vi "校准设置页.vi"() -> ()   [LabVIEW 2016, in "斯坦道氨氮.lvlib"]
uses:
  <vilib>/Analysis/6fits.llb/Curve Fitting Criteria.ctl
  <vilib>/Analysis/NI_AALPro.lvlib
  <vilib>/ptbypt/NI_PtbyPt.lvlib
panel:
  out "刷新时间":string
  out "校准状态":T1(ring)
  out "模型刷新":bool
  in  "校准按钮":T2(radio)
  in  "校准导入":bool
  in  "辅助计算":bool
  in  "曲线模型":T3={"标液浓度1"=0.0, "测量吸光度1"=0.0, "样品1启用"=FALSE, "标液浓度2"=0.0, "测量吸光度2"=0.0, "样品2启用"=FALSE, "标液浓度3"=0.0, "测量吸光度3"=0.0, "样品3启用"=FALSE, "标液浓度4"=0.0, "测量吸光度4"=0.0, "样品4启用"=FALSE, "标液浓度5"=0.0, "测量吸光度5"=0.0, "样品5启用"=FALSE, "模型"=enum."线性", "精度"=4.0, "XY图"=[], "拟合公式"="", "r^2"=0.0, "标样一校准时间"=timestamp(0 s since 1904-01-01), "标样二校准时间"=timestamp(0 s since 1904-01-01), "标样三校准时间"=timestamp(0 s since 1904-01-01), "标样四校准时间"=timestamp(0 s since 1904-01-01), "标样五校准时间"=timestamp(0 s since 1904-01-01), "二次方程"={"c"=0.0, "x"=0.0, "x^2"=0.0}, "标定时间"=timestamp(0 s since 1904-01-01)} {"标定时间" format="%<%m/%d/%y %H:%M:%S>T"; "标样五校准时间" format="%<%m/%d/%y %H:%M:%S>T"; "标样四校准时间" format="%<%m/%d/%y %H:%M:%S>T"; "标样三校准时间" format="%<%m/%d/%y %H:%M:%S>T"; "标样二校准时间" format="%<%m/%d/%y %H:%M:%S>T"; "标样一校准时间" format="%<%m/%d/%y %H:%M:%S>T"; "r^2" format="%.7f"; "测量吸光度5" format="%#.6f"; "测量吸光度4" format="%#.6f"; "测量吸光度3" format="%#.6f"; "测量吸光度2" format="%#.6f"; "测量吸光度1" format="%#.6f"}
  in  "测量模式":T4(ring)
  in  "参数下拉列表":u16(ring)
  in  "量程下拉列表":enum16{"低量程", "高量程"}(ring)
  # "校准时间"
  # "标液浓度"
  # "吸光值显示"
  # "标液一"
  # "标液二"
  # "标液三"
  # "零点"
  # "跨度"
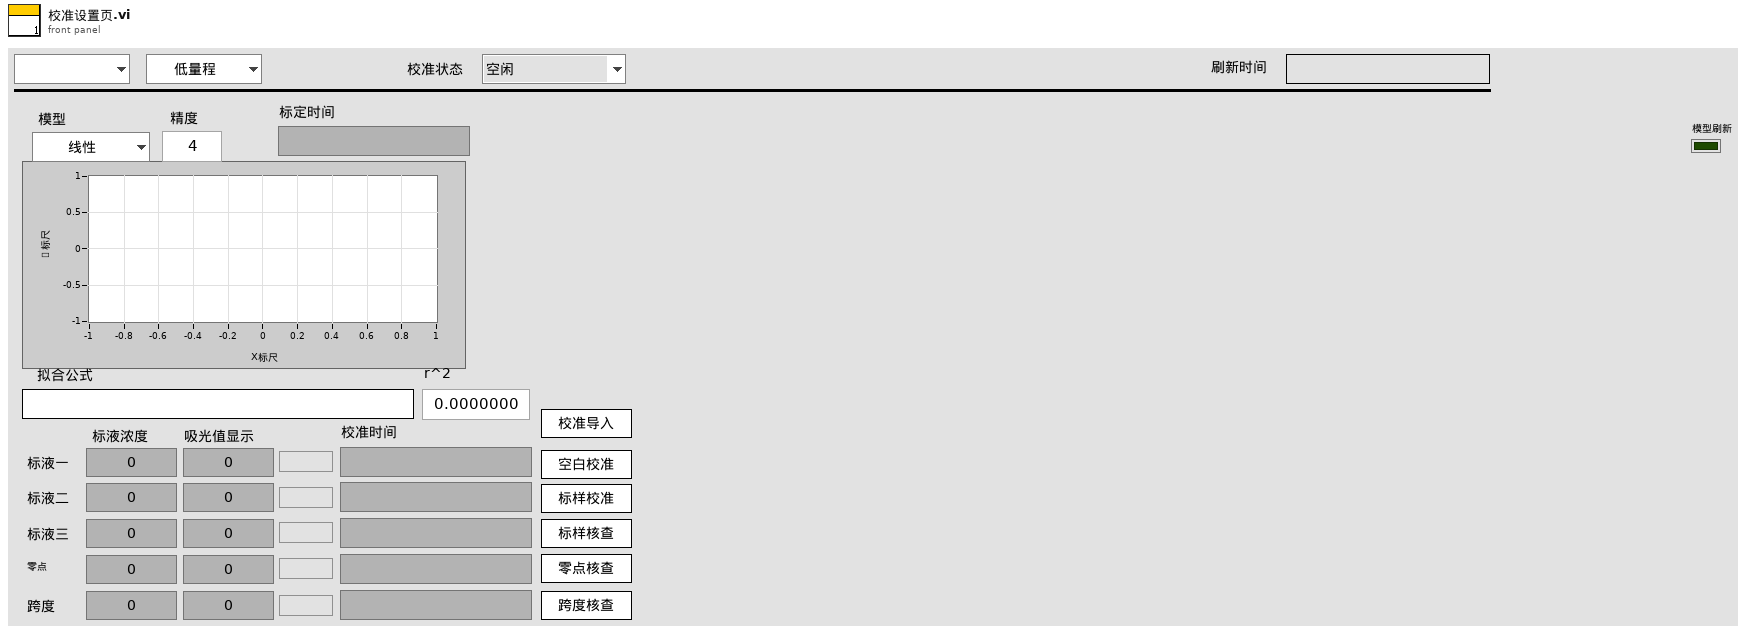
[diagram p1: front panel]
types:
  T1 = enum16{"空闲", "初始化", "校准启动", "校准运行中", "测试结束", "获取校准数据", "填充校准数据", "流程结束"}
  T2 = enum32{"未选择", "空白校准", "标样校准", "标样核查", "零点核查", "跨度核查"}
  T3 = cluster{"标液浓度1":dbl, "测量吸光度1":dbl, "样品1启用":bool, "标液浓度2":dbl, "测量吸光度2":dbl, "样品2启用":bool, "标液浓度3":dbl, "测量吸光度3":dbl, "样品3启用":bool, "标液浓度4":dbl, "测量吸光度4":dbl, "样品4启用":bool, "标液浓度5":dbl, "测量吸光度5":dbl, "样品5启用":bool, "模型":enum32{"线性", "多项式"}, "精度":dbl, "XY图":cluster{"X Values":dbl[], "Y Values":dbl[]}[], "拟合公式":string, "r^2":dbl, "标样一校准时间":timestamp, "标样二校准时间":timestamp, "标样三校准时间":timestamp, "标样四校准时间":timestamp, "标样五校准时间":timestamp, "二次方程":cluster{"c":dbl, "x":dbl, "x^2":dbl}, "标定时间":timestamp}
  T4 = enum16{"跨度核查", "水样测量", "零点核查", "标样核查", "加标回收", "快捷测试", "空白校准", "标样校准"}
  T5 = typedef "LVStringsAndValuesArrayTypeDef_U16.ctl" = cluster{"String":string, "Value":u16}[]
  T6 = enum8{"Enabled", "Disabled", "Disabled and Grayed Out"}
  T7 = cluster{"标液浓度1":dbl, "测量吸光度1":dbl, "样品1启用":bool, "标液浓度2":dbl, "测量吸光度2":dbl, "样品2启用":bool, "标液浓度3":dbl, "测量吸光度3":dbl, "样品3启用":bool, "标液浓度4":dbl, "测量吸光度4":dbl, "样品4启用":bool, "标液浓度5":dbl, "测量吸光度5":dbl, "样品5启用":bool, "模型":enum32{"线性", "多项式"}, "精度":dbl, "XY图":cluster{"X Values":dbl[], "Y Values":dbl[]}[], "拟合公式":string, "r^2":dbl, "标样一校准时间":timestamp, "标样二校准时间":timestamp, "标样三校准时间":timestamp, "标样四校准时间":timestamp, "标样五校准时间":timestamp, "二次方程":cluster{"c":dbl, "x":dbl, "x^2":dbl}, "标定时间":timestamp}[][]
  T8 = typedef "NI_AALPro.lvlib/Curve Fitting Criteria.ctl" = u16
  T9 = enum32{"Bad", "Idle", "Run top level", "Running"}
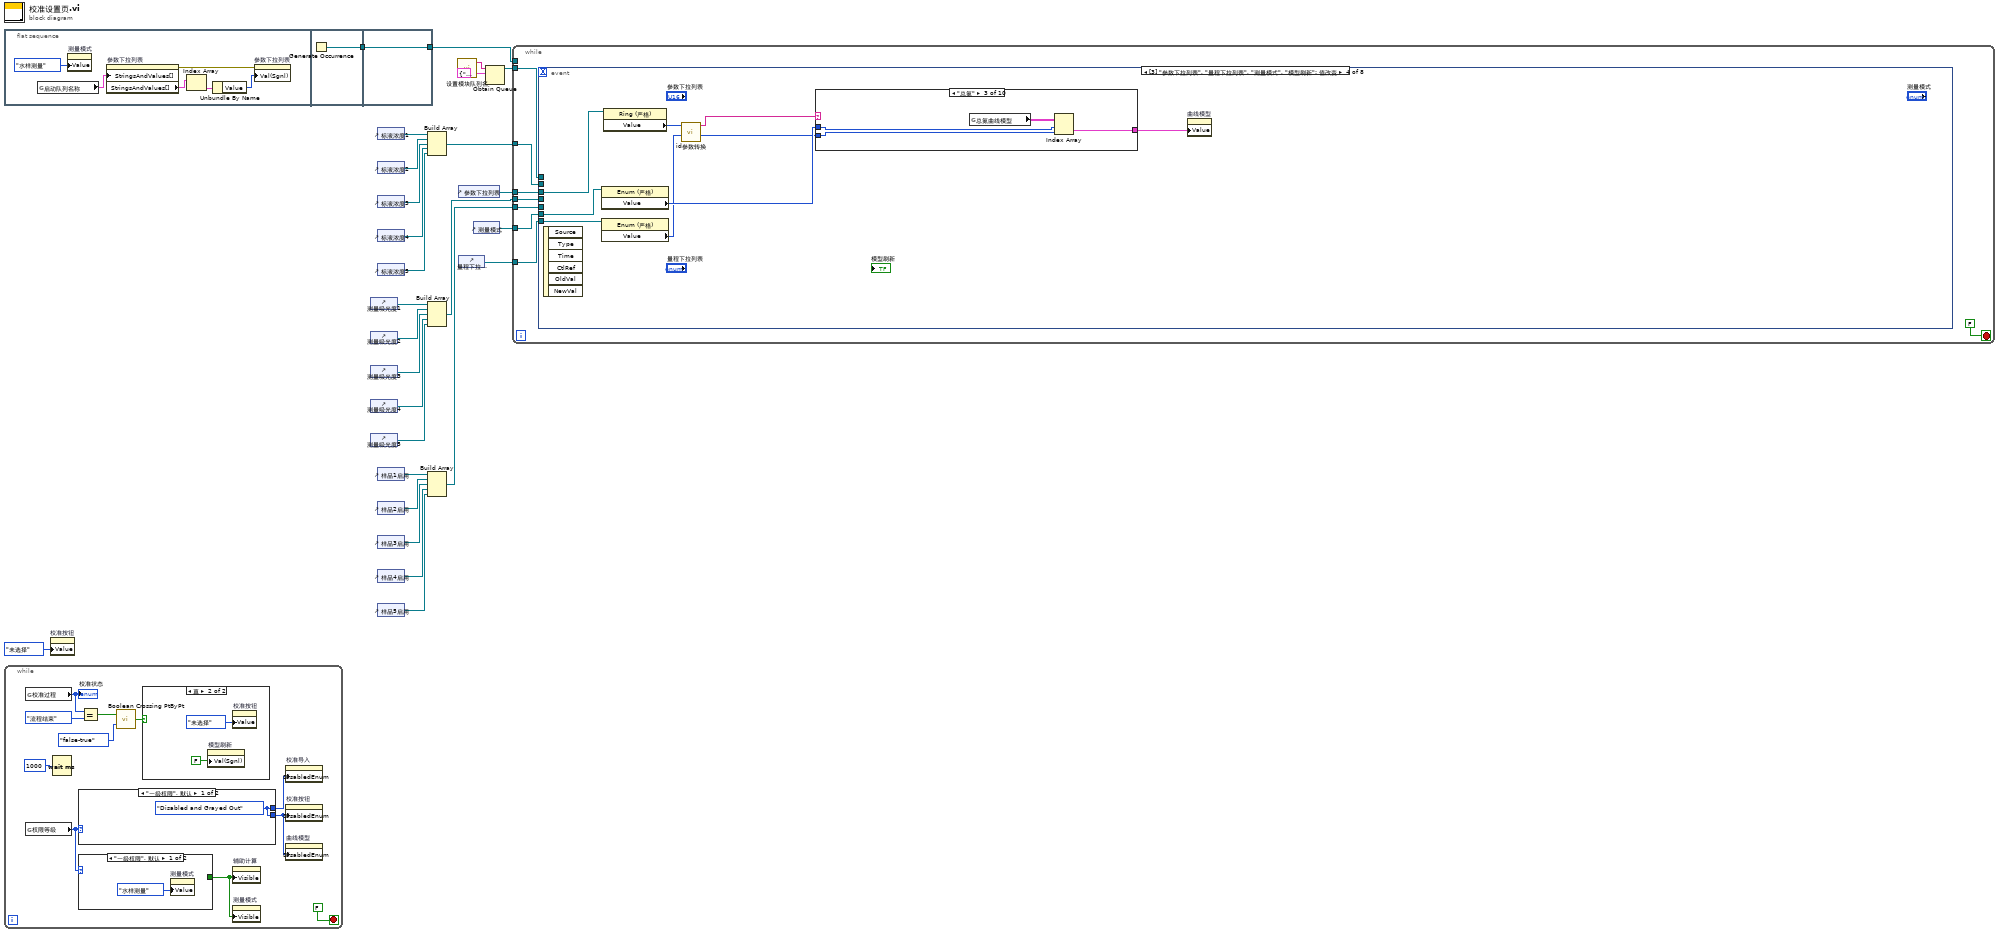
[diagram p0: block diagram]
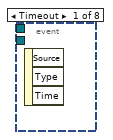
[diagram p2: hidden frame]
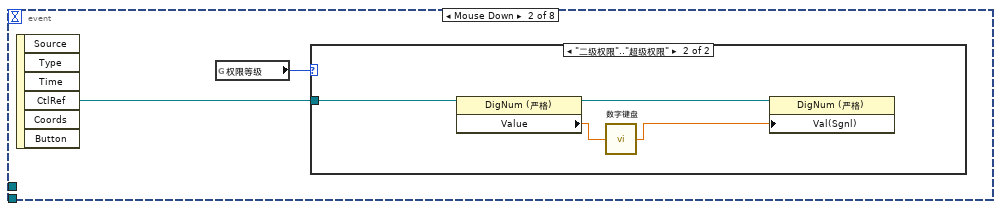
[diagram p3: hidden frame]
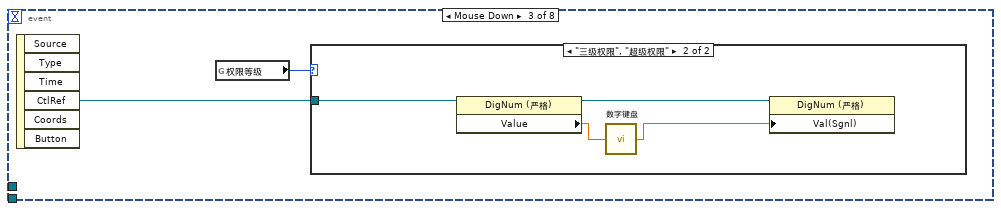
[diagram p5: hidden frame]
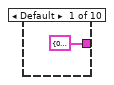
[diagram p7: hidden frame]
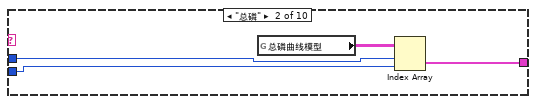
[diagram p8: hidden frame]
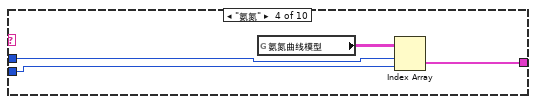
[diagram p9: hidden frame]
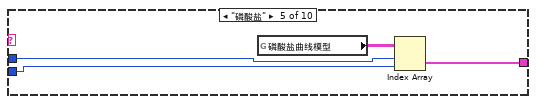
[diagram p10: hidden frame]
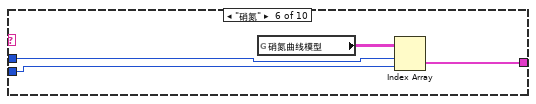
[diagram p11: hidden frame]
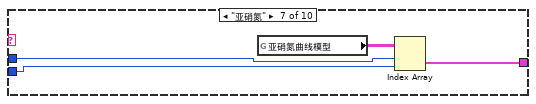
[diagram p12: hidden frame]
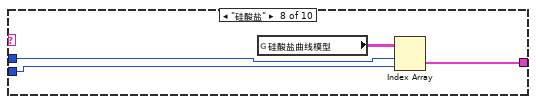
[diagram p13: hidden frame]
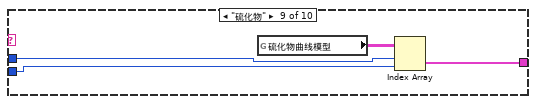
[diagram p14: hidden frame]
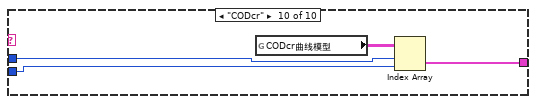
[diagram p15: hidden frame]
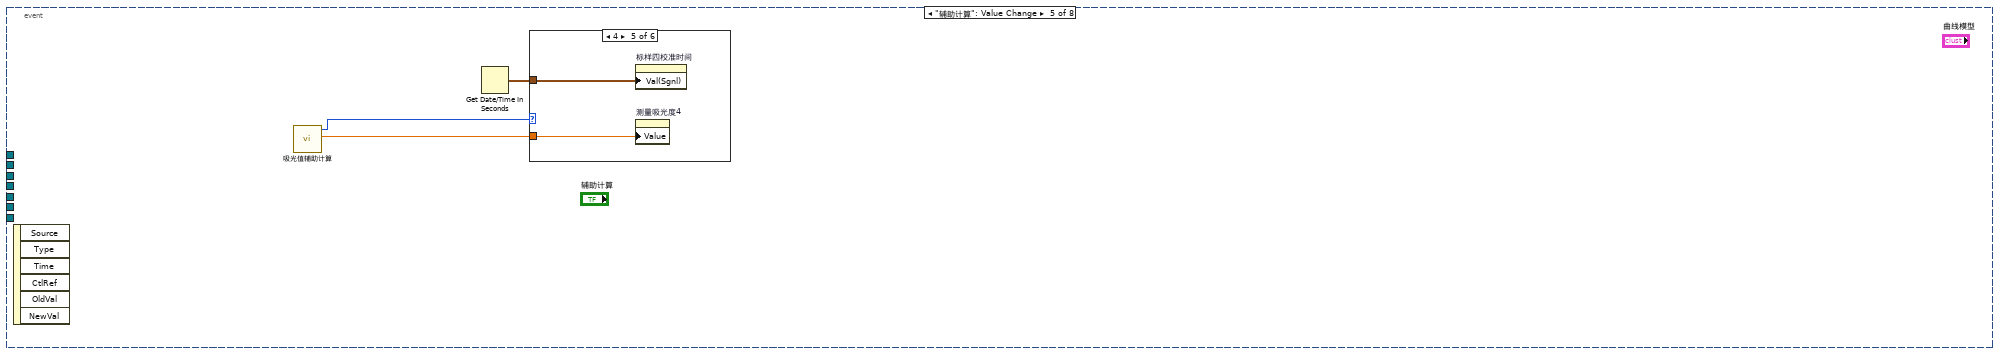
[diagram p16: hidden frame]
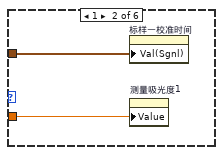
[diagram p18: hidden frame]
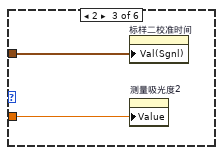
[diagram p19: hidden frame]
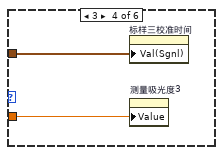
[diagram p20: hidden frame]
diagram:
  n1 = flat-sequence {
    tunnel: [w34] -> w27
    tunnel: [w35] -> w26
    tunnel: w27 -> [w35]
    frame #0 {
      n2 = global read "总磷总氮断电保存全局变量.vi" "启动队列名称"() -> (w29:cluster{"String":string, "Value":u16}[])
      n3 = property on="测量模式" class="Enum (严格)"("Value"=T4."水样测量" ("测量模式")) -> ()  [unwired: 2 in, 2 out]
      n4 = property on="参数下拉列表" class="Ring (严格)"("StringsAndValues[]"=w29) -> (error out=w32:errorcluster, "StringsAndValues[]"=w30:T5)  [unwired: 2 in, 1 out]
      n5 = Index Array(array=w30) -> (element=w31:cluster{"String":string, "Value":u16})  [unwired: 1 in]
      n6 = Unbundle By Name(w31) -> ("Value"=w33:u16)
      n7 = property on="参数下拉列表" class="Ring (严格)"(error in=w32, "Val(Sgnl)"=w33) -> ()  [unwired: 1 in, 2 out]
    }
    frame #1 {
      n8 = Generate Occurrence() -> (w34:refnum<k4>)
    }
    frame #2 {
    }
  }
  n9 = while {
    stop <- FALSE stop-if-true
    n10 = global read "VAR总磷总氮全局变量.vi" "校准过程"() -> (w37:T1)
    "校准状态" <- w37
    n11 = global read "VAR总磷总氮全局变量.vi" "权限等级"() -> (w43:enum16{"一级权限", "二级权限", "三级权限", "超级权限"})
    n12 = Wait (ms)(milliseconds to wait=u32 1000 ("等待时间（毫秒）")) -> ()  [unwired: 1 out]
    n13 = case shown="\"一级权限\", 默认" w43 {
      tunnel: [w51 w52] -> w41
      tunnel: [w51 w52] -> w44
      frame "一级权限", Default {
        w51 = T6."Disabled and Grayed Out" ("禁用")
      }
      frame "二级权限".."超级权限" {
        w52 = T6."Enabled" ("禁用")
      }
    }
    n14 = case shown="\"一级权限\", 默认" w43 {
      tunnel: [_ TRUE ("可见")] -> w42
      frame "一级权限", Default {
        n15 = property on="测量模式" class="Enum (严格)"("Value"=T4."水样测量" ("测量模式")) -> ()  [unwired: 2 in, 2 out]
      }
      frame "三级权限", "超级权限" {
      }
    }
    n16 = Equal?(x=w37, y=T1."流程结束" ("校准过程")) -> (x = y?=w40:bool)
    n17 = call <vilib>:"Boolean Crossing PtByPt.vi"("direction"=enum16{"either", "false-true", "true-false"}."false-true", "input"=w40) -> ("crossing"=w38:bool)  [unwired: 1 in]
    n18 = case shown="真" w38 {
      frame False {
      }
      frame True {
        n19 = property on="模型刷新" class="Bool (严格)"("Val(Sgnl)"=FALSE ("值(信号)")) -> ()  [unwired: 2 in, 2 out]
        n20 = property on="校准按钮" class="RadioBtnsControl (严格)"("Value"=T2."未选择" ("校准按钮")) -> ()  [unwired: 2 in, 2 out]
      }
    }
    n21 = property on="辅助计算" class="Bool"("Visible"=w42) -> ()  [unwired: 2 in, 2 out]
    n22 = property on="测量模式" class="Enum (严格)"("Visible"=w42) -> ()  [unwired: 2 in, 2 out]
    n23 = property on="校准导入" class="Bool"("DisabledEnum"=w44) -> ()  [unwired: 2 in, 2 out]
    n24 = property on="校准按钮" class="RadioBtnsControl (严格)"("DisabledEnum"=w41) -> ()  [unwired: 2 in, 2 out]
    n25 = property on="曲线模型" class="Clust (严格)"("DisabledEnum"=w41) -> ()  [unwired: 2 in, 2 out]
  }
  n26 = property on="校准按钮" class="RadioBtnsControl (严格)"("Value"=T2."未选择" ("校准按钮")) -> ()  [unwired: 2 in, 2 out]
  n27 = control-ref of="测量吸光度1"() -> (w15:refnum<vi>)
  n28 = control-ref of="测量吸光度2"() -> (w16:refnum<vi>)
  n29 = control-ref of="测量吸光度3"() -> (w17:refnum<vi>)
  n30 = control-ref of="测量吸光度4"() -> (w18:refnum<vi>)
  n31 = control-ref of="测量吸光度5"() -> (w19:refnum<vi>)
  n32 = control-ref of="标液浓度1"() -> (w13:refnum<vi>)
  n33 = control-ref of="标液浓度2"() -> (w12:refnum<vi>)
  n34 = control-ref of="标液浓度3"() -> (w11:refnum<vi>)
  n35 = control-ref of="标液浓度4"() -> (w10:refnum<vi>)
  n36 = control-ref of="标液浓度5"() -> (w9:refnum<vi>)
  n37 = control-ref of="样品1启用"() -> (w25:refnum<vi>)
  n38 = control-ref of="样品2启用"() -> (w24:refnum<vi>)
  n39 = control-ref of="样品3启用"() -> (w23:refnum<vi>)
  n40 = control-ref of="样品4启用"() -> (w22:refnum<vi>)
  n41 = control-ref of="样品5启用"() -> (w21:refnum<vi>)
  n42 = Build Array(w13, w12, w11, w10, w9) -> (w8:refnum<vi>[])
  n43 = Build Array(w15, w16, w17, w18, w19) -> (w14:refnum<vi>[])
  n44 = Build Array(w25, w24, w23, w22, w21) -> (w20:refnum<vi>[])
  n45 = call "设置模块队列名.vi"() -> ("Msg"=w6:string)  [unwired: 5 in]
  n46 = control-ref of="参数下拉列表"() -> (w3:refnum<vi>)
  n47 = control-ref of="量程下拉列表"() -> (w1:refnum<vi>)
  n48 = control-ref of="测量模式"() -> (w2:refnum<vi>)
  n49 = Obtain Queue(name (unnamed)=w6, element data type=cluster{"命令":string, "data":variant} {"命令"="", "data"=variant}) -> (queue out=w5:refnum<queue>)  [unwired: 3 in, 2 out]
  n50 = while {
    tunnel: w26 -> [_]
    tunnel: w3 -> [w59]
    tunnel: w20 -> [w58]
    tunnel: w14 -> [w57]
    tunnel: w8 -> [w56]
    tunnel: w2 -> [w55]
    tunnel: w1 -> [w54]
    tunnel: w5 -> [w53]
    stop <- FALSE stop-if-true
    n51 = event shown="[3] \"参数下拉列表\", \"量程下拉列表\", \"测量模式\", \"模型刷新\": 值改变" {
      selector: _ -> [_ _ _ _ _ _ _ _]
      dyn-events: _ -> [_ _ _ _ _ _ _ _]
      timeout: _ -> [_ _ _ _ _ _ _ _]
      tunnel: w59 -> [_ _ _ w79 _ w143 w189 w278]
      tunnel: w58 -> [_ _ _ _ _ _ w193 _]
      tunnel: w57 -> [_ _ _ _ _ _ w192 _]
      tunnel: w56 -> [_ _ _ _ _ _ w191 _]
      tunnel: w55 -> [_ _ _ w77 _ w141 w187 w273]
      tunnel: w54 -> [_ _ _ w76 _ w139 w185 w277]
      tunnel: w53 -> [_ _ _ _ _ _ _ w279]
      event Timeout {
        n52 = event-data() -> ()  [unwired: 1 in, 3 out]
      }
      event "曲线模型.标液浓度1", "曲线模型.标液浓度2", "曲线模型.标液浓度3", "曲线模型.标液浓度4", "曲线模型.标液浓度5", "曲线模型.精度": Mouse Down {
        n53 = event-data() -> ("CtlRef"=w62:refnum<vi>)  [unwired: 1 in, 5 out]
        n54 = global read "VAR总磷总氮全局变量.vi" "权限等级"() -> (w61:enum16{"一级权限", "二级权限", "三级权限", "超级权限"})
        n55 = case shown="\"二级权限\"..\"超级权限\"" w61 {
          tunnel: w62 -> [_ w66]
          frame "一级权限", Default {
          }
          frame "二级权限".."超级权限" {
            n56 = property class="DigNum (严格)"(reference=w66) -> (reference out=w64:refnum<vi>, "Value"=w65:dbl)  [unwired: 1 in, 1 out]
            n57 = call "数字键盘.vi"("OldNumber"=w65) -> ("NewNumber"=w63:dbl)
            n58 = property class="DigNum (严格)"(reference=w64, "Val(Sgnl)"=w63) -> ()  [unwired: 1 in, 2 out]
          }
        }
      }
      event "曲线模型.测量吸光度1", "曲线模型.测量吸光度2", "曲线模型.测量吸光度3", "曲线模型.测量吸光度4", "曲线模型.测量吸光度5": Mouse Down {
        n59 = event-data() -> ("CtlRef"=w68:refnum<vi>)  [unwired: 1 in, 5 out]
        n60 = global read "VAR总磷总氮全局变量.vi" "权限等级"() -> (w67:enum16{"一级权限", "二级权限", "三级权限", "超级权限"})
        n61 = case shown="\"三级权限\", \"超级权限\"" w67 {
          tunnel: w68 -> [_ w72]
          frame "一级权限", Default {
          }
          frame "三级权限", "超级权限" {
            n62 = property class="DigNum (严格)"(reference=w72) -> (reference out=w70:refnum<vi>, "Value"=w71:dbl)  [unwired: 1 in, 1 out]
            n63 = call "数字键盘.vi"("OldNumber"=w71) -> ("NewNumber"=w69:dbl)
            n64 = property class="DigNum (严格)"(reference=w70, "Val(Sgnl)"=w69) -> ()  [unwired: 1 in, 2 out]
          }
        }
      }
      event "参数下拉列表", "量程下拉列表", "测量模式", "模型刷新": Value Change {
        n65 = event-data() -> ()  [unwired: 1 in, 6 out]
        n66 = property class="Enum (严格)"(reference=w77) -> ("Value"=w74:T4)  [unwired: 1 in, 2 out]
        n67 = property class="Enum (严格)"(reference=w76) -> ("Value"=w73:enum16{"低量程", "高量程"})  [unwired: 1 in, 2 out]
        n68 = property class="Ring (严格)"(reference=w79) -> ("Value"=w80:u16)  [unwired: 1 in, 2 out]
        n69 = call "id参数转换.vi"("id"=w80) -> ("table输出"=w78:string)  [unwired: 9 in, 1 out]
        n70 = case shown="\"总氮\"" w78 {
          tunnel: w73 -> [_ w84 w89 w91 w95 w99 w103 w107 w111 w115]
          tunnel: w74 -> [_ w85 w88 w92 w96 w100 w104 w108 w112 w116]
          tunnel: [T3 {"标液浓度1"=0.0, "测量吸光度1"=0.0, "样品1启用"=FALSE, "标液浓度2"=0.0, "测量吸光度2"=0.0, "样品2启用"=FALSE, "标液浓度3"=0.0, "测量吸光度3"=0.0, "样品3启用"=FALSE, "标液浓度4"=0.0, "测量吸光度4"=0.0, "样品4启用"=FALSE, "标液浓度5"=0.0, "测量吸光度5"=0.0, "样品5启用"=FALSE, "模型"=enum."线性", "精度"=0.0, "XY图"=[], "拟合公式"="", "r^2"=0.0, "标样一校准时间"=timestamp(0 s since 1904-01-01), "标样二校准时间"=timestamp(0 s since 1904-01-01), "标样三校准时间"=timestamp(0 s since 1904-01-01), "标样四校准时间"=timestamp(0 s since 1904-01-01), "标样五校准时间"=timestamp(0 s since 1904-01-01), "二次方程"={"c"=0.0, "x"=0.0, "x^2"=0.0}, "标定时间"=timestamp(0 s since 1904-01-01)} ("总磷曲线模型") w82 w86 w90 w94 w98 w102 w106 w110 w114] -> w75
          frame Default {
          }
          frame "总磷" {
            n71 = global read "校准数据全局变量.vi" "总磷曲线模型"() -> (w83:T7)
            n72 = Index Array(array=w83, index (row)=w85, index (col)=w84) -> (element=w82:T3)
          }
          frame "总氮" {
            n73 = global read "校准数据全局变量.vi" "总氮曲线模型"() -> (w87:T7)
            n74 = Index Array(array=w87, index (row)=w88, index (col)=w89) -> (element=w86:T3)
          }
          frame "氨氮" {
            n75 = global read "校准数据全局变量.vi" "氨氮曲线模型"() -> (w93:T7)
            n76 = Index Array(array=w93, index (row)=w92, index (col)=w91) -> (element=w90:T3)
          }
          frame "磷酸盐" {
            n77 = global read "校准数据全局变量.vi" "磷酸盐曲线模型"() -> (w97:T7)
            n78 = Index Array(array=w97, index (row)=w96, index (col)=w95) -> (element=w94:T3)
          }
          frame "硝氮" {
            n79 = global read "校准数据全局变量.vi" "硝氮曲线模型"() -> (w101:T7)
            n80 = Index Array(array=w101, index (row)=w100, index (col)=w99) -> (element=w98:T3)
          }
          frame "亚硝氮" {
            n81 = global read "校准数据全局变量.vi" "亚硝氮曲线模型"() -> (w105:T7)
            n82 = Index Array(array=w105, index (row)=w104, index (col)=w103) -> (element=w102:T3)
          }
          frame "硅酸盐" {
            n83 = global read "校准数据全局变量.vi" "硅酸盐曲线模型"() -> (w109:T7)
            n84 = Index Array(array=w109, index (row)=w108, index (col)=w107) -> (element=w106:T3)
          }
          frame "硫化物" {
            n85 = global read "校准数据全局变量.vi" "硫化物曲线模型"() -> (w113:T7)
            n86 = Index Array(array=w113, index (row)=w112, index (col)=w111) -> (element=w110:T3)
          }
          frame "CODcr" {
            n87 = global read "校准数据全局变量.vi" "CODcr曲线模型"() -> (w117:T7)
            n88 = Index Array(array=w117, index (row)=w116, index (col)=w115) -> (element=w114:T3)
          }
        }
        n89 = property on="曲线模型" class="Clust (严格)"("Value"=w75) -> ()  [unwired: 2 in, 2 out]
      }
      event "辅助计算": Value Change {
        n90 = event-data() -> ()  [unwired: 1 in, 6 out]
        n91 = call "吸光值辅助计算.vi"() -> ("X"=w119:dbl, "吸光值导出"=w120:u16)  [unwired: 10 in]
        n92 = Get Date/Time In Seconds() -> (seconds since 1Jan1904=w118:timestamp)
        n93 = case shown="4" w120 {
          tunnel: w119 -> [_ w122 w124 w126 w128 w130]
          tunnel: w118 -> [_ w121 w123 w125 w127 w129]
          frame 0, Default {
          }
          frame 1 {
            n94 = property on="标样一校准时间" class="AbsTime (严格)"("Val(Sgnl)"=w121) -> ()  [unwired: 2 in, 2 out]
            n95 = property on="测量吸光度1" class="DigNum (严格)"("Value"=w122) -> ()  [unwired: 2 in, 2 out]
          }
          frame 2 {
            n96 = property on="标样二校准时间" class="AbsTime (严格)"("Val(Sgnl)"=w123) -> ()  [unwired: 2 in, 2 out]
            n97 = property on="测量吸光度2" class="DigNum (严格)"("Value"=w124) -> ()  [unwired: 2 in, 2 out]
          }
          frame 3 {
            n98 = property on="标样三校准时间" class="AbsTime (严格)"("Val(Sgnl)"=w125) -> ()  [unwired: 2 in, 2 out]
            n99 = property on="测量吸光度3" class="DigNum (严格)"("Value"=w126) -> ()  [unwired: 2 in, 2 out]
          }
          frame 4 {
            n100 = property on="标样四校准时间" class="AbsTime (严格)"("Val(Sgnl)"=w127) -> ()  [unwired: 2 in, 2 out]
            n101 = property on="测量吸光度4" class="DigNum (严格)"("Value"=w128) -> ()  [unwired: 2 in, 2 out]
          }
          frame 5 {
            n102 = property on="标样五校准时间" class="AbsTime (严格)"("Val(Sgnl)"=w129) -> ()  [unwired: 2 in, 2 out]
            n103 = property on="测量吸光度5" class="DigNum (严格)"("Value"=w130) -> ()  [unwired: 2 in, 2 out]
          }
        }
      }
      event "校准导入": Value Change {
        n104 = event-data() -> ()  [unwired: 1 in, 6 out]
        n105 = property class="Enum (严格)"(reference=w141) -> ("Value"=w140:T4)  [unwired: 1 in, 2 out]
        n106 = property class="Enum (严格)"(reference=w139) -> ("Value"=w138:enum16{"低量程", "高量程"})  [unwired: 1 in, 2 out]
        n107 = property class="Ring (严格)"(reference=w143) -> ("Value"=w142:u16)  [unwired: 1 in, 2 out]
        n108 = property on="二次方程" class="Clust (严格)"() -> ("Value"=w132:cluster{"c":dbl, "x":dbl, "x^2":dbl})  [unwired: 2 in, 2 out]
        n109 = Unbundle By Name(w132) -> ("x^2"=w134:dbl, "x"=w135:dbl, "c"=w136:dbl)
        n110 = Bundle By Name(cluster=cluster{"X^2":dbl, "X":dbl, "b":dbl} {"X^2"=0.0, "X"=0.0, "b"=0.0} ("公式"), "X^2"=w134, "X"=w135, "b"=w136) -> (w131:cluster{"X^2":dbl, "X":dbl, "b":dbl})
        n111 = global read "VAR总磷总氮全局变量.vi" "权限等级"() -> (w137:enum16{"一级权限", "二级权限", "三级权限", "超级权限"})
        n112 = case shown="\"一级权限\", 默认" w137 {
          tunnel: w142 -> [w152 w183]
          tunnel: w140 -> [w151 w182]
          tunnel: w138 -> [w150 w181]
          tunnel: w131 -> [w144 _]
          frame "一级权限", Default {
            n113 = Cluster To Array(cluster=w144) -> (array=w149:dbl[])
            n114 = Add Array Elements(numeric array=w149) -> (sum=w148:dbl)
            n115 = Equal To 0?(x=w148) -> (x = 0?=w146:bool)
            n116 = Not A Number/Path/Refnum?(number/path/refnum=w148) -> (NaN/Path/Refnum?=w147:bool)
            n117 = Or(x=w146, y=w147) -> (x .or. y?=w145:bool)
            n118 = case shown="假" w145 {
              tunnel: w152 -> [w158 _]
              tunnel: w151 -> [w157 _]
              tunnel: w150 -> [w156 _]
              tunnel: w144 -> [w153 _]
              frame False {
                n119 = Two Button Dialog(message="请再一次确认是否导入" ("消息")) -> (T button?=w154:bool)  [unwired: 2 in]
                n120 = case shown="真" w154 {
                  tunnel: w158 -> [_ w160]
                  tunnel: w157 -> [_ w166]
                  tunnel: w156 -> [_ w159]
                  tunnel: w153 -> [_ w161]
                  frame False {
                  }
                  frame True {
                    n121 = for {
                      N: 8 -> [_]
                      tunnel: w160 -> [w172]
                      tunnel: w166 -> [_]
                      tunnel: w159 -> [w171]
                      shift-right: [w170] -> w164
                      shift-left: errorcluster {"status"=FALSE, "code"=0, "source"=""} ("error out") -> [w167]
                      tunnel: w161 -> [w168]
                      i -> [w169]
                      n122 = call "总磷总氮公式写入.vi"("公式"=w168, "error in (no error)"=w167, "量程"=w171, "测量模式"=w169, "测量参数"=w172) -> ("error out"=w170:errorcluster)  [unwired: 6 in]
                    }
                    n123 = case shown="无错误" w164 {
                      tunnel: ["写入成功" "写入失败"] -> w165
                      tunnel: w160 -> [w176 _]
                      tunnel: w159 -> [w175 _]
                      frame No Error {
                        n124 = Get Date/Time In Seconds() -> (seconds since 1Jan1904=w177:timestamp)
                        n125 = property on="标定时间" class="AbsTime (严格)"("Val(Sgnl)"=w177) -> (error out=w173:errorcluster)  [unwired: 2 in, 1 out]
                        n126 = property on="曲线模型" class="Clust (严格)"(error in=w173) -> ("Value"=w174:T3)  [unwired: 1 in, 2 out]
                        n127 = call "校准记录.vi"("曲线模型"=w174, "量程"=w175, "校准参数"=w176) -> ()  [unwired: 8 in, 1 out]
                      }
                      frame Error {
                      }
                    }
                    n128 = One Button Dialog(message=w165) -> ()  [unwired: 1 in, 1 out]
                  }
                }
              }
              frame True {
                n129 = One Button Dialog(message="校准数据异常，请重新校准！" ("消息")) -> ()  [unwired: 1 in, 1 out]
              }
            }
          }
          frame "三级权限", "超级权限" {
            n130 = call "公式复合写入.vi"("量程下拉列表"=w181, "测量模式"=w182, "参数下拉列表"=w183) -> ()  [unwired: 9 in]
          }
        }
      }
      event "曲线模型": Value Change {
        n131 = event-data() -> ()  [unwired: 1 in, 6 out]
        n132 = flat-sequence {
          tunnel: w193 -> [w213]
          tunnel: w192 -> [w211]
          tunnel: w191 -> [w209]
          tunnel: [w196] -> w190
          tunnel: w189 -> [w196]
          tunnel: [w195] -> w188
          tunnel: w187 -> [w195]
          tunnel: [w194] -> w186
          tunnel: w185 -> [w194]
          tunnel: w190 -> [w227]
          tunnel: w188 -> [w223]
          tunnel: w186 -> [w222]
          frame #0 {
            w205 = T8 0 items=["最小二乘", "最小绝对残差", "Bisquare"] ("method")
            n133 = for {
              tunnel: w213 -> [w219] mode=indexing
              tunnel: [w218] -> w212 mode=indexing
              tunnel: w211 -> [w217] mode=indexing
              tunnel: [w216] -> w210 mode=indexing
              tunnel: w209 -> [w215] mode=indexing
              tunnel: [w214] -> w208 mode=indexing
              n134 = property class="DigNum (严格)"(reference=w215) -> ("Value"=w214:dbl)  [unwired: 1 in, 2 out]
              n135 = property class="DigNum (严格)"(reference=w217) -> ("Value"=w216:dbl)  [unwired: 1 in, 2 out]
              n136 = property class="Bool (严格)"(reference=w219) -> ("Value"=w218:bool)  [unwired: 1 in, 2 out]
            }
            n137 = property on="模型" class="Enum (严格)"() -> ("Value"=w207:enum32{"线性", "多项式"})  [unwired: 2 in, 2 out]
            n138 = property on="精度" class="DigNum (严格)"() -> ("Value"=w206:dbl)  [unwired: 2 in, 2 out]
            n139 = call "线性公式.vi"("精度"=w206, "模型"=w207, "method"=w205, "启用"=w212, "监测浓度"=w210, "标液浓度"=w208) -> ("Polynomial Coefficients 2"=w201:dbl[], "XY图"=w202:cluster{"X Values":dbl[], "Y Values":dbl[]}[], "r^2"=w203:dbl, "拟合方程"=w204:string)  [unwired: 2 in]
            n140 = property on="拟合公式" class="Str"("Value"=w204) -> ()  [unwired: 2 in, 2 out]
            n141 = property on="r^2" class="DigNum (严格)"("Value"=w203) -> ()  [unwired: 2 in, 2 out]
            n142 = property on="XY图" class="XYGraph (严格)"("Value"=w202) -> ()  [unwired: 2 in, 2 out]
            n143 = Index Array(array=w201) -> (element #1=w200:dbl, element #2=w199:dbl, element #3=w198:dbl)  [unwired: 3 in]
            n144 = Bundle("slope"=w200, "slope"=w199, "slope"=w198) -> (w197:cluster{"slope":dbl, "slope":dbl, "slope":dbl})  [unwired: 1 in]
            n145 = property on="二次方程" class="Clust (严格)"("Value"=w197) -> ()  [unwired: 2 in, 2 out]
          }
          frame #1 {
            n146 = property class="Enum (严格)"(reference=w223) -> ("Value"=w220:T4)  [unwired: 1 in, 2 out]
            n147 = property class="Enum (严格)"(reference=w222) -> ("Value"=w221:enum16{"低量程", "高量程"})  [unwired: 1 in, 2 out]
            n148 = property class="Ring (严格)"(reference=w227) -> ("Value"=w226:u16)  [unwired: 1 in, 2 out]
            n149 = call "id参数转换.vi"("id"=w226) -> ("table输出"=w225:string)  [unwired: 9 in, 1 out]
            n150 = property on="曲线模型" class="Clust (严格)"() -> ("Value"=w224:T3)  [unwired: 2 in, 2 out]
            n151 = case shown="\"总氮\"" w225 {
              tunnel: w224 -> [_ w232 w237 w239 w243 w248 w253 w258 w263 w269]
              tunnel: w221 -> [_ w230 w236 w240 w244 w249 w254 w259 w264 w270]
              tunnel: w220 -> [_ w231 w235 w241 w245 w250 w255 w260 w265 w271]
              frame Default {
              }
              frame "总磷" {
                n152 = global read "校准数据全局变量.vi" "总磷曲线模型"() -> (w228:T7)
                n153 = Replace Array Subset(array=w228, new element=w232, index (row)=w231, index (col)=w230) -> (w229:T7)
                n154 = global write "校准数据全局变量.vi" "总磷曲线模型"(w229) -> ()
              }
              frame "总氮" {
                n155 = global read "校准数据全局变量.vi" "总氮曲线模型"() -> (w234:T7)
                n156 = Replace Array Subset(array=w234, new element=w237, index (row)=w235, index (col)=w236) -> (w233:T7)
                n157 = global write "校准数据全局变量.vi" "总氮曲线模型"(w233) -> ()
              }
              frame "氨氮" {
                n158 = global read "校准数据全局变量.vi" "氨氮曲线模型"() -> (w242:T7)
                n159 = Replace Array Subset(array=w242, new element=w239, index (row)=w241, index (col)=w240) -> (w238:T7)
                n160 = global write "校准数据全局变量.vi" "氨氮曲线模型"(w238) -> ()
              }
              frame "磷酸盐" {
                n161 = global read "校准数据全局变量.vi" "磷酸盐曲线模型"() -> (w247:T7)
                n162 = Replace Array Subset(array=w247, new element=w243, index (row)=w245, index (col)=w244) -> (w246:T7)
                n163 = global write "校准数据全局变量.vi" "磷酸盐曲线模型"(w246) -> ()
              }
              frame "硝氮" {
                n164 = global read "校准数据全局变量.vi" "硝氮曲线模型"() -> (w252:T7)
                n165 = Replace Array Subset(array=w252, new element=w248, index (row)=w250, index (col)=w249) -> (w251:T7)
                n166 = global write "校准数据全局变量.vi" "硝氮曲线模型"(w251) -> ()
              }
              frame "亚硝氮" {
                n167 = global read "校准数据全局变量.vi" "亚硝氮曲线模型"() -> (w257:T7)
                n168 = Replace Array Subset(array=w257, new element=w253, index (row)=w255, index (col)=w254) -> (w256:T7)
                n169 = global write "校准数据全局变量.vi" "亚硝氮曲线模型"(w256) -> ()
              }
              frame "硅酸盐" {
                n170 = global read "校准数据全局变量.vi" "硅酸盐曲线模型"() -> (w262:T7)
                n171 = Replace Array Subset(array=w262, new element=w258, index (row)=w260, index (col)=w259) -> (w261:T7)
                n172 = global write "校准数据全局变量.vi" "硅酸盐曲线模型"(w261) -> ()
              }
              frame "硫化物" {
                n173 = global read "校准数据全局变量.vi" "硫化物曲线模型"() -> (w267:T7)
                n174 = Replace Array Subset(array=w267, new element=w263, index (row)=w265, index (col)=w264) -> (w266:T7)
                n175 = global write "校准数据全局变量.vi" "硫化物曲线模型"(w266) -> ()
              }
              frame "CODcr" {
                n176 = global read "校准数据全局变量.vi" "CODcr曲线模型"() -> (w272:T7)
                n177 = Replace Array Subset(array=w272, new element=w269, index (row)=w271, index (col)=w270) -> (w268:T7)
                n178 = global write "校准数据全局变量.vi" "CODcr曲线模型"(w268) -> ()
              }
            }
          }
          frame #2 {
            n179 = call "校准数据写入配置文件.vi"() -> ()  [unwired: 11 in, 1 out]
          }
        }
        n180 = Format Date/Time String() -> (date/time string=→"刷新时间":string)  [unwired: 3 in]
      }
      event "校准按钮": Value Change {
        n181 = event-data() -> ("NewVal"=w274:T2)  [unwired: 1 in, 5 out]
        n182 = Not Equal?(x=w274, y=T2."未选择") -> (x != y?=w275:bool)
        n183 = case shown="真" w275 {
          tunnel: w279 -> [_ _]
          tunnel: w278 -> [_ w290]
          tunnel: w277 -> [_ w289]
          tunnel: w274 -> [_ w284]
          tunnel: w273 -> [_ w288]
          frame False {
          }
          frame True {
            n184 = property class="Enum (严格)"(reference=w288) -> ("Value"=w282:T4)  [unwired: 1 in, 2 out]
            n185 = property class="Enum (严格)"(reference=w289) -> ("Value"=w281:enum16{"低量程", "高量程"})  [unwired: 1 in, 2 out]
            n186 = property class="Ring (严格)"(reference=w290) -> ("Value"=w283:u16)  [unwired: 1 in, 2 out]
            n187 = vi-ref "校准流程.vi"() -> (w285:refnum<vi>)
            n188 = local read "曲线模型"() -> (w280:T3)
            n189 = property class="VI"(reference=w285) -> ("Name"=w286:string, "Exec.State"=w287:T9)  [unwired: 1 in, 2 out]
            n190 = case shown="\"Bad\", 默认" w287 {
              tunnel: w286 -> [_ w303]
              tunnel: w284 -> [_ w296]
              tunnel: w283 -> [_ w295]
              tunnel: w282 -> [_ w294]
              tunnel: w281 -> [_ w293]
              tunnel: w280 -> [_ w292]
              frame "Bad", Default {
                n191 = One Button Dialog(message="正在校准，请在校准完成后操作！" ("消息")) -> ()  [unwired: 1 in, 1 out]
              }
              frame "Idle" {
                n192 = Open VI Reference(type specifier VI Refnum (for type only)=refnum<vi> refnum, vi path=w303, options=128 ("选项")) -> (vi reference=w301:refnum<vi>, error out=w300:errorcluster)  [unwired: 3 in]
                n193 = call-by-ref "开始异步调用"(reference=w301, error in=w300, "校准模式"=w296, "参数下拉列表"=w295, "测量模式"=w294, "量程下拉列表"=w293, "曲线模型"=w292) -> (reference out=w298:refnum<vi>, error out=w299:errorcluster)  [unwired: 11 in]
                n194 = Close Reference(reference=w298, error in (no error)=w299) -> ()  [unwired: 1 out]
              }
            }
          }
        }
      }
    }
  }
